vi "132CameraPortal20210521.vi"() -> ()   [LabVIEW 2019]
doc: "This example shows how to load VIs into a subpanel control, and display them on the front panel of a host VI."
panel:
  in  "Ring":u16(ring) items=["fisrt VI", "second VI"]
  in  "Path for second VI":path=path "Right Click >> Browse for second VI"
  in  "Path for first VI":path=path "Right Click >> Browse for first VI"
  in  "stop":bool
  in  "Change subVI":bool
  # "Overview: This example shows how to load VIs into a subpanel control, and display them on the front panel of a host VI.\nRequirements: LabVIEW 2012 (or compatible)\nInstructions:\n1. Negative to the paths of first and second  subVI  in the path controls. \n2. Run the VI and the Sub Panel will display the front panel of subVI.\n3. Toggle the \"Change subVI\" button to toggle between the front panels of the two VIs."
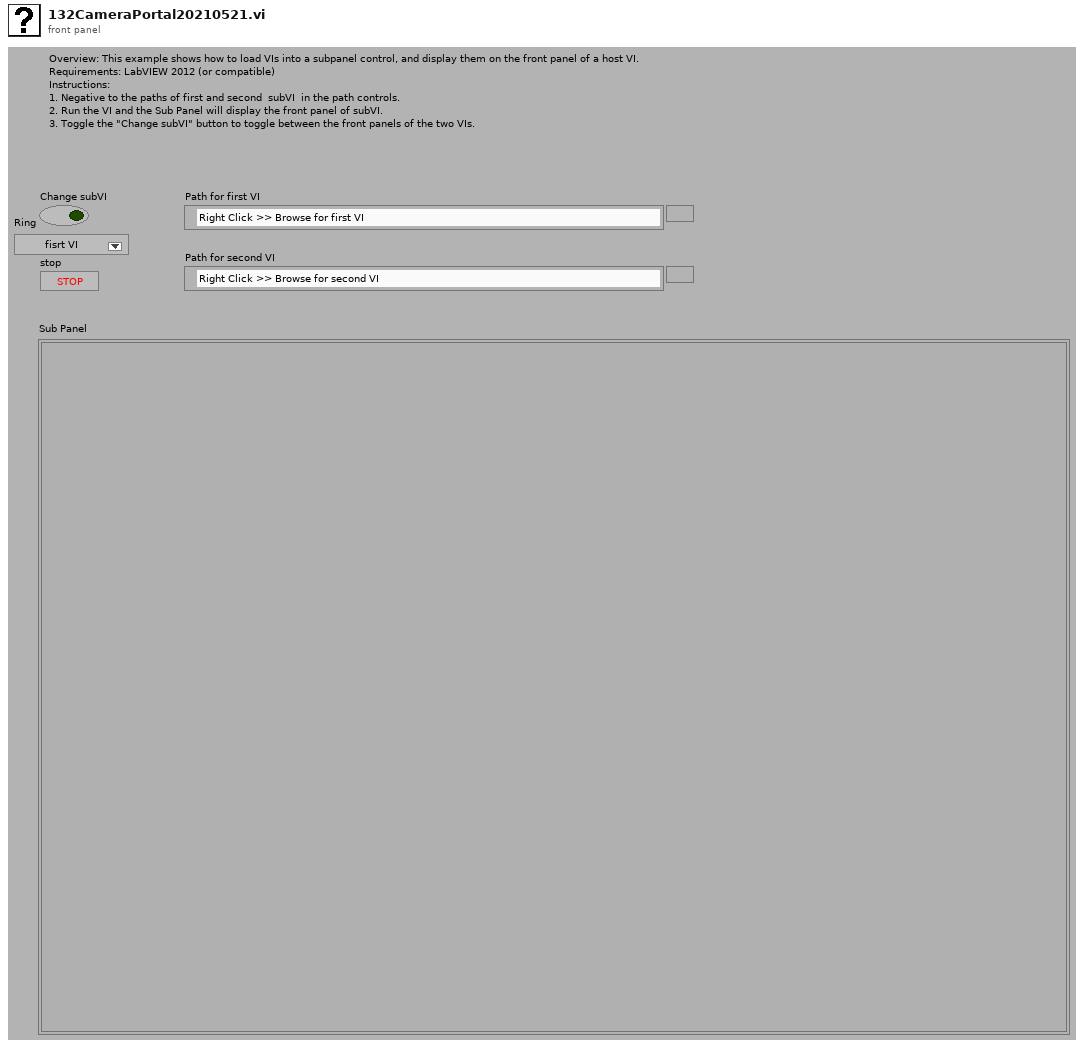
[diagram p1: front panel]
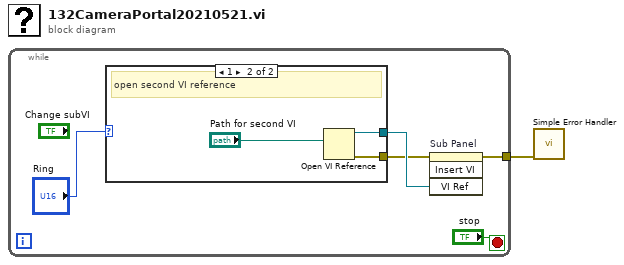
[diagram p0: block diagram]
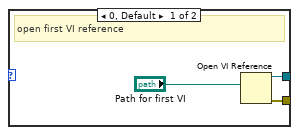
[diagram p2: hidden frame]
diagram:
  n1 = while {
    tunnel: [w3] -> w1
    stop <- "stop" stop-if-true
    n2 = case shown="1" "Ring" {
      tunnel: [w9 w12] -> w6
      tunnel: [w7 w10] -> w4
      frame 0, Default {
        # "open first VI reference"
        n3 = Open VI Reference(vi path="Path for first VI") -> (vi reference=w9:refnum<vi>, error out=w7:errorcluster)  [unwired: 5 in]
      }
      frame 1 {
        # "open second VI reference"
        n4 = Open VI Reference(vi path="Path for second VI") -> (vi reference=w12:refnum<vi>, error out=w10:errorcluster)  [unwired: 5 in]
      }
    }
    n5 = invoke on="Sub Panel" class="SubPanel" method="Insert VI"(error in=w4, "VI Ref"=w6) -> (error out=w3:errorcluster)  [unwired: 2 in, 3 out]
  }
  n6 = call <vilib>:"Simple Error Handler.vi"("error in (no error)"=w1) -> ()  [unwired: 4 in, 5 out]
